vi "Write Map.vi"(8 "error in":errorcluster, 10 "Map":T1, 11 "Ballard ARINC-429 Tx Execution Unit in":refnum<class "Ballard ARINC-429 Tx Execution Unit.lvclass">) -> (0 "error out":errorcluster, 3 "Ballard ARINC-429 Tx Execution Unit out":refnum<class "Ballard ARINC-429 Tx Execution Unit.lvclass">)   [LabVIEW 2020, in "Ballard ARINC 429 Engine.lvlib" / "Implementation.lvlib" / "Ballard ARINC-429 Tx Execution Unit.lvclass"]
uses:
  Ballard ARINC-429 Tx Execution Unit.lvclass
  Shared/Map of Values Indexes to Channel and Label Indexes.ctl
  Ballard ARINC-429 Tx Execution Unit.lvclass/Ballard ARINC-429 Tx Execution Unit.ctl
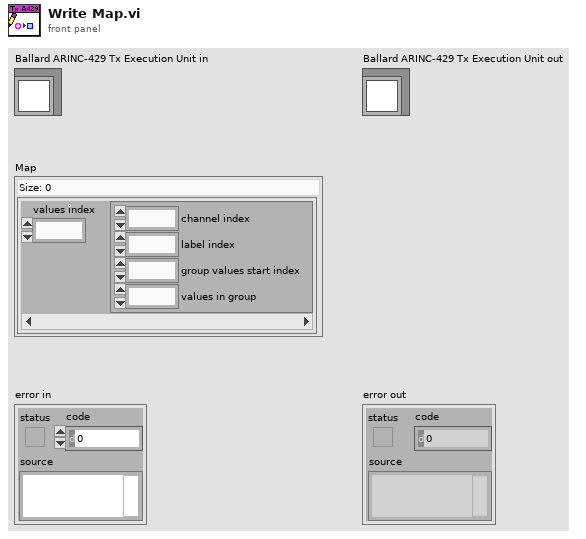
[diagram p1: front panel]
types:
  T1 = typedef "Map of Values Indexes to Channel and Label Indexes.ctl" = map{i32, cluster{"channel index":i32, "label index":i32, "group values start index":i32, "values in group":i32}}
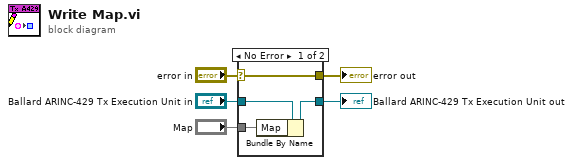
[diagram p0: block diagram]
diagram:
  n1 = case shown="No Error" "error in" {
    selector: "error in" -> [w9 w10]
    tunnel: [w9 w10] -> w4
    tunnel: [w6 w11] -> w2
    tunnel: "Ballard ARINC-429 Tx Execution Unit in" -> [w8 w11]
    tunnel: "Map" -> [w7 _]
    frame No Error {
      n2 = Bundle By Name(cluster=w8, "Map"=w7) -> (w6:refnum<class "Ballard ARINC-429 Tx Execution Unit.lvclass">)
    }
    frame Error {
    }
  }
  "error out" <- w4
  "Ballard ARINC-429 Tx Execution Unit out" <- w2
